vi "test_riccat_01i.vi"() -> (3 "All Tests Passed":bool)   [LabVIEW 2019]
uses:
  <vilib>/Analysis/Matrix/Datatypes/RealMatrix.ctl
  <vilib>/Rock Robotics/WPI/ThirdParty/JAS_Junk/TrajLib/Trajectory_Library.lvlib
  <vilib>/Analysis/Matrix/NI_Matrix.lvlib
panel:
  out "Eigenvalues":cdb[](array[numeric])
  out "error out":errorcluster
  out "Error":bool
  out "Iterations":i32
  out "Elapsed \nTime MS":dbl
  out "ZERO":T1
  out "X  Answer":T1
  in  "R":T1=[[0.25]]
  in  "Q":T1=[[1.0, 0.0, 0.0, 0.0], [0.0, 0.0, 0.0, 0.0], [0.0, 0.0, 0.0, 0.0], [0.0, 0.0, 0.0, 0.0]]
  in  "B":T1=[[0.0], [0.0], [0.0], [1.0]]
  in  "A":T1=[[0.5, 1.0, 0.0, 0.0], [0.0, 0.0, 1.0, 0.0], [0.0, 0.0, 0.0, 1.0], [0.0, 0.0, 0.0, 0.0]]
  # "Test 1: non-invertible A\n  // Example 2 of \"On the Numerical Solution of the Discrete-Time Algebraic\n  // Riccati Equation\""
  # "int n1 = 4, m1 = 1;"
  # "Example = F"
  # "MatrixXd A1(n1, n1), B1(n1, m1), Q1(n1, n1), R1(m1, m1);"
  # "A1 << 0.5, 1, 0, 0, \n          0, 0, 1, 0, \n          0, 0, 0, 1, \n          0, 0, 0, 0;"
  # "B1 << 0, \n        0, \n        0, \n        1;"
  # "Example G1"
  # "Example H"
  # "Solution weight ??"
  # "Q1 << 1, 0, 0, 0, \n        0, 0, 0, 0, \n        0, 0, 0, 0, \n        0, 0, 0, 0;"
  # "Example G2"
  # "Cost ??"
  # "R1 << 0.25;"
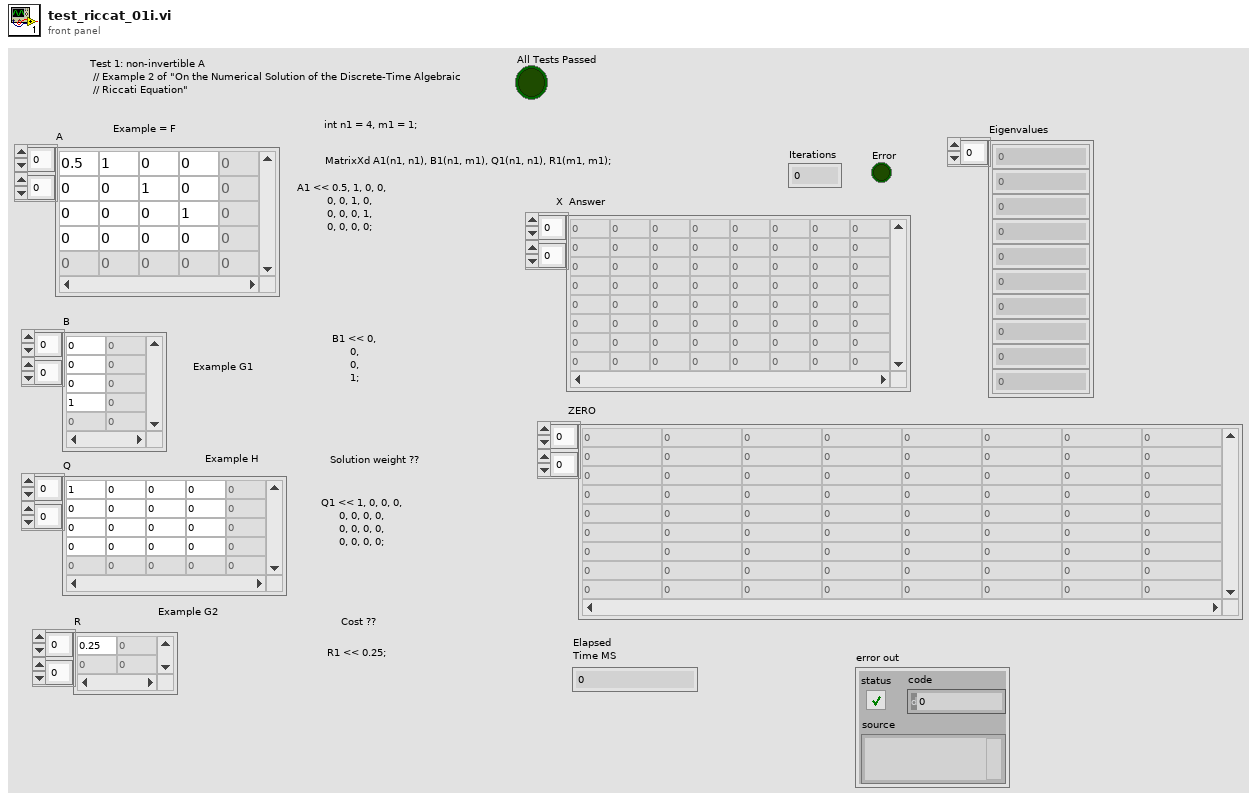
[diagram p1: front panel]
types:
  T1 = typedef "NI_Matrix.lvlib/RealMatrix.ctl" = dbl[][]
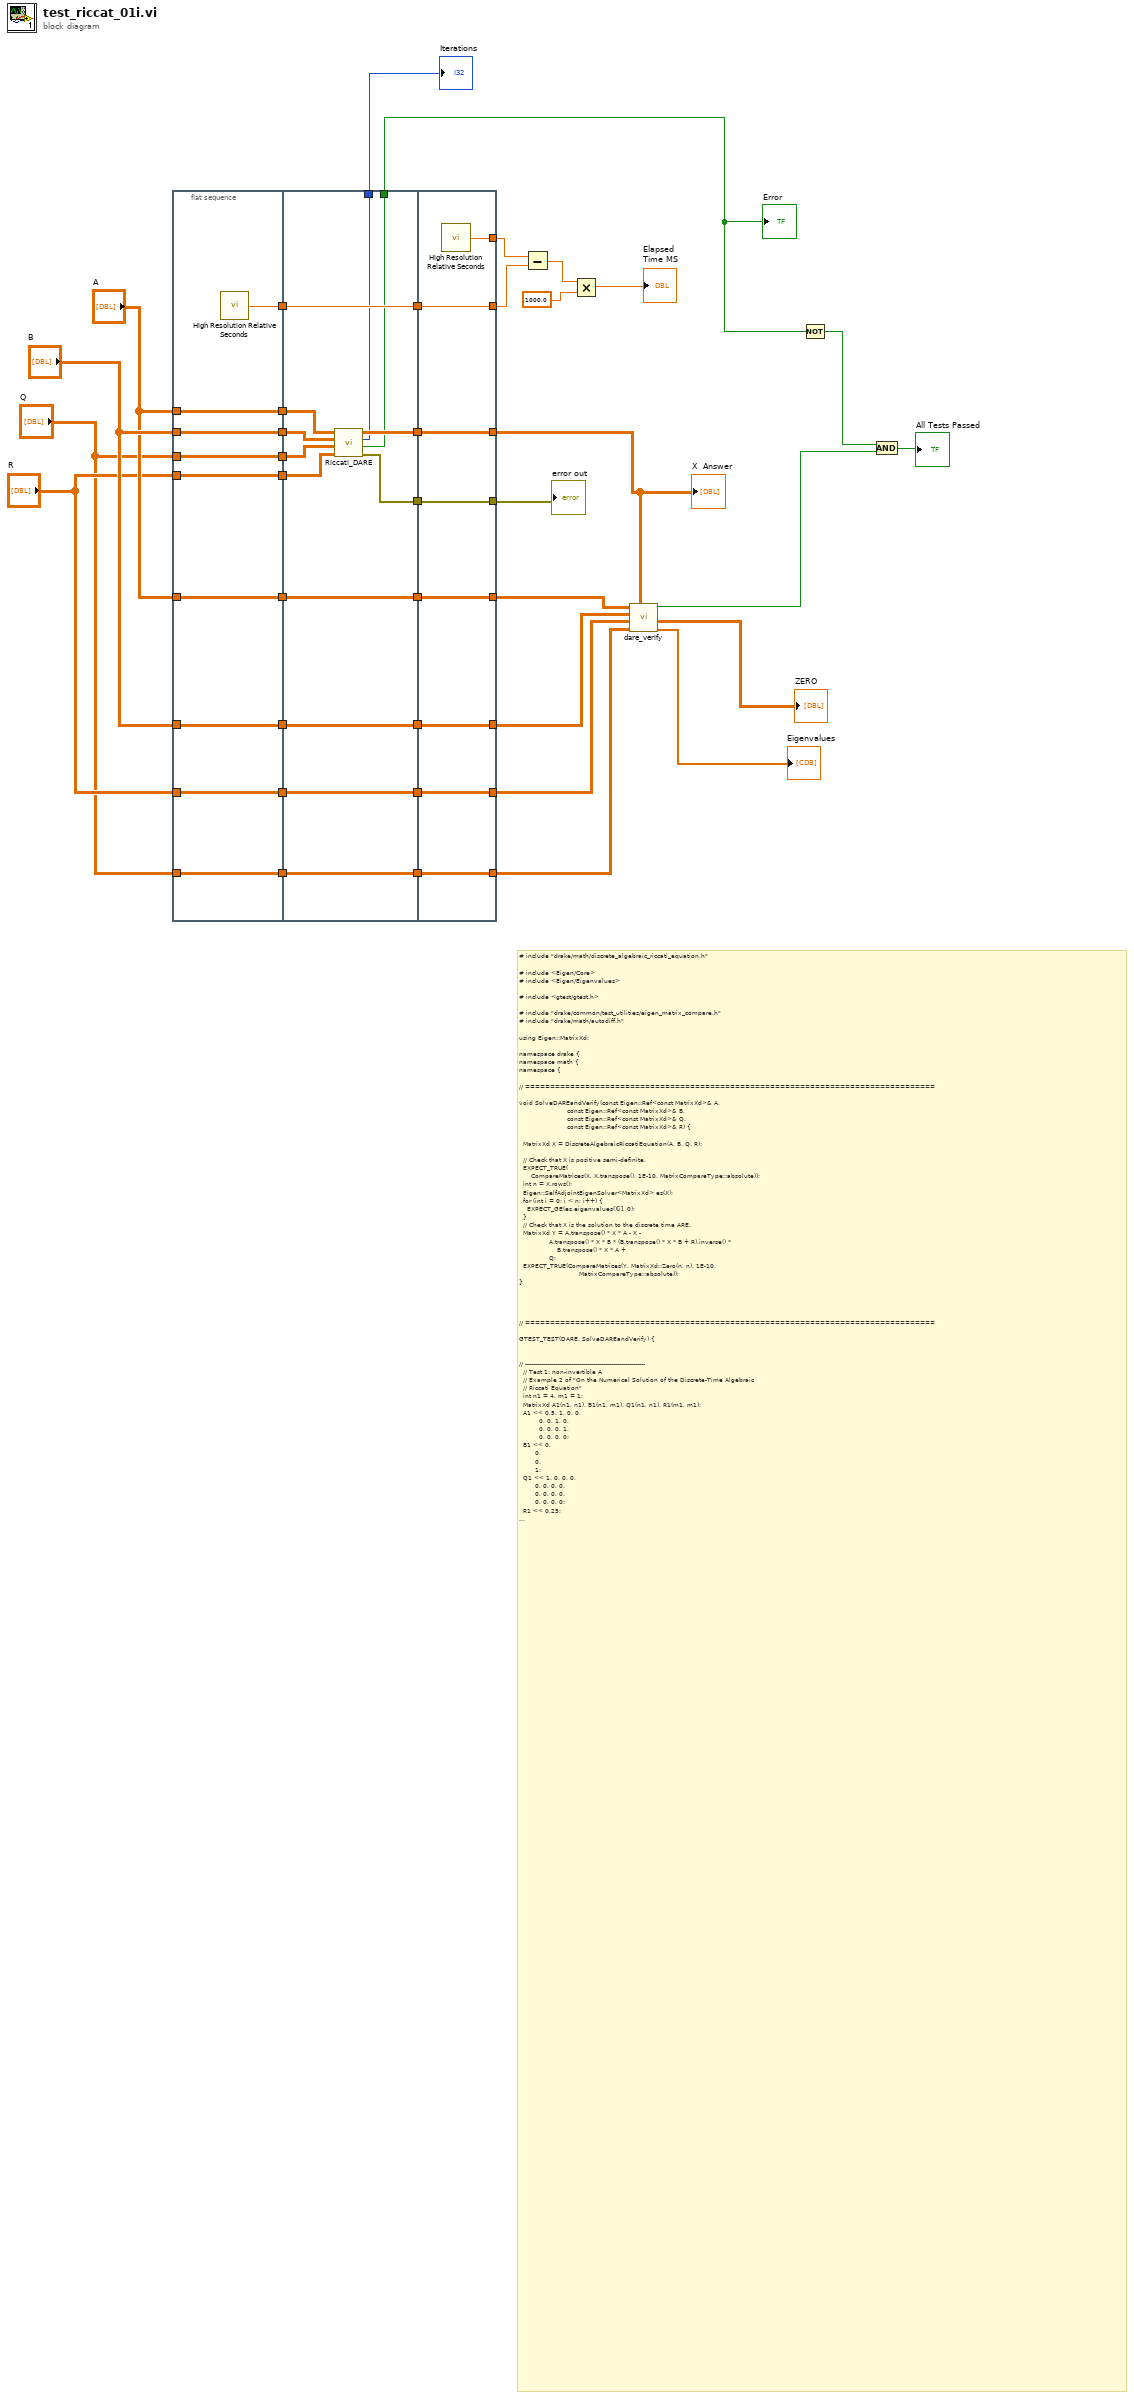
[diagram p0: block diagram]
diagram:
  # "# include \"drake/math/discrete_algebraic_riccati_equation.h\"\n\n# include <Eigen/Core>\n# include <Eigen/Eigenvalues>\n\n# include <gtest/gtest.h>\n\n# include \"drake/common/test_utilities/eigen_matrix_compare.h\"\n# include \"drake/math/autodiff.h\"\n\nusing Eigen::MatrixXd;\n\nnamespace drake {\nnamespace math {\nnamespace {\n\n// ==================================================================================\n\nvoid SolveDAREandVerify(const Eigen::Ref<const MatrixXd>& A,\n                        const Eigen::Ref<const MatrixXd>& B,\n                        const Eigen::Ref<const MatrixXd>& Q,\n                        const Eigen::Ref<const MatrixXd>& R) {\n\n  MatrixXd X = DiscreteAlgebraicRiccatiEquation(A, B, Q, R);\n\n  // Check that X is positive semi-definite.\n  EXPECT_TRUE(\n      CompareMatrices(X, X.transpose(), 1E-10, MatrixCompareType::absolute));\n  int n = X.rows();\n  Eigen::SelfAdjointEigenSolver<MatrixXd> es(X);\n  for (int i = 0; i < n; i++) {\n    EXPECT_GE(es.eigenvalues()[i], 0);\n  }\n  // Check that X is the solution to the discrete time ARE.\n  MatrixXd Y = A.transpose() * X * A - X -\n               A.transpose() * X * B * (B.transpose() * X * B + R).inverse() *\n                   B.transpose() * X * A +\n               Q;\n  EXPECT_TRUE(CompareMatrices(Y, MatrixXd::Zero(n, n), 1E-10,\n                              MatrixCompareType::absolute));\n}\n\n\n\n\n// ==================================================================================\n\nGTEST_TEST(DARE, SolveDAREandVerify) {\n\n\n// ------------------------------------------------------------\n  // Test 1: non-invertible A\n  // Example 2 of \"On the Numerical Solution of the Discrete-Time Algebraic\n  // Riccati Equation\"\n  int n1 = 4, m1 = 1;\n  MatrixXd A1(n1, n1), B1(n1, m1), Q1(n1, n1), R1(m1, m1);\n  A1 << 0.5, 1, 0, 0, \n          0, 0, 1, 0, \n          0, 0, 0, 1, \n          0, 0, 0, 0;\n  B1 << 0, \n        0, \n        0, \n        1;\n  Q1 << 1, 0, 0, 0, \n        0, 0, 0, 0, \n        0, 0, 0, 0, \n        0, 0, 0, 0;\n  R1 << 0.25;\n  SolveDAREandVerify(A1, B1, Q1, R1);\n// ------------------------------------------------------------\n  // Test 2: invertible A\n  int n2 = 2, m2 = 1;\n  MatrixXd A2(n2, n2), B2(n2, m2), Q2(n2, n2), R2(m2, m2);\n  A2 << 1, 1, 0, 1;\n  B2 << 0, 1;\n  Q2 << 1, 0, 0, 0;\n  R2 << 0.3;\n  SolveDAREandVerify(A2, B2, Q2, R2);\n\n// ------------------------------------------------------------\n  // Test 3: the first generalized eigenvalue of (S,T) is stable\n  int n3 = 2, m3 = 1;\n  MatrixXd A3(n3, n3), B3(n3, m3), Q3(n3, n3), R3(m3, m3);\n  A3 << 0, 1, 0, 0;\n  B3 << 0, 1;\n  Q3 << 1, 0, 0, 1;\n  R3 << 1;\n  SolveDAREandVerify(A3, B3, Q3, R3);\n\n// ------------------------------------------------------------\n  // Test 4: A = B = Q = R = I_2 (2-by-2 identity matrix)\n  int n4 = 2, m4 = 2;\n  MatrixXd A4(n4, n4), B4(n4, m4), Q4(n4, n4), R4(m4, m4);\n  A4 << 1, 0, 0, 1;\n  B4 << 1, 0, 0, 1;\n  Q4 << 1, 0, 0, 1;\n  R4 << 1, 0, 0, 1;\n  SolveDAREandVerify(A4, B4, Q4, R4);\n\n// ------------------------------------------------------------\n}\n}  // namespace\n}  // namespace math\n}  // namespace drake"
  n1 = flat-sequence {
    tunnel: "B" -> [w42]
    tunnel: "A" -> [w43]
    tunnel: "B" -> [w44]
    tunnel: "Q" -> [w45]
    tunnel: "A" -> [w46]
    tunnel: "R" -> [w47]
    tunnel: [w47] -> w38
    tunnel: [w46] -> w37
    tunnel: [w45] -> w36
    tunnel: [w44] -> w35
    tunnel: [w43] -> w34
    tunnel: [w42] -> w33
    tunnel: "R" -> [w41]
    tunnel: [w41] -> w26
    tunnel: "Q" -> [w40]
    tunnel: [w40] -> w24
    tunnel: [w39] -> w18
    tunnel: w38 -> [w60]
    tunnel: w37 -> [w58]
    tunnel: w36 -> [w57]
    tunnel: w35 -> [w56]
    tunnel: w34 -> [w55]
    tunnel: w33 -> [w54]
    tunnel: [w59] -> w32
    tunnel: [w55] -> w31
    tunnel: [w54] -> w30
    tunnel: [w53] -> w27
    tunnel: w26 -> [w53]
    tunnel: w24 -> [w52]
    tunnel: [w52] -> w23
    tunnel: [w51] -> w19
    tunnel: w18 -> [w51]
    tunnel: [w50] -> w14
    tunnel: [w49] -> w13
    tunnel: [w48] -> w12
    tunnel: [w66] -> w8
    tunnel: [w67] -> w9
    tunnel: [w68] -> w10
    tunnel: w32 -> [w68]
    tunnel: w31 -> [w67]
    tunnel: w30 -> [w66]
    tunnel: [w65] -> w7
    tunnel: w27 -> [w65]
    tunnel: [w64] -> w6
    tunnel: w23 -> [w64]
    tunnel: [w63] -> w21
    tunnel: [w62] -> w20
    tunnel: w19 -> [w62]
    tunnel: w12 -> [w61]
    tunnel: [w61] -> w11
    frame #0 {
      n2 = call <vilib>:"High Resolution Relative Seconds.vi"() -> ("relative seconds"=w39:dbl)
    }
    frame #1 {
      n3 = call <vilib>:"Riccati_DARE.vi"("R"=w60, "Q"=w57, "B"=w56, "A"=w58) -> ("error out"=w48:errorcluster, "Error"=w49:bool, "Iterations"=w50:i32, "Answer"=w59:T1)  [unwired: 4 in]
    }
    frame #2 {
      n4 = call <vilib>:"High Resolution Relative Seconds.vi"() -> ("relative seconds"=w63:dbl)
    }
  }
  n5 = Subtract(x=w21, y=w20) -> (x-y=w17:dbl)
  n6 = Multiply(x=w17, y=1000.0) -> (x*y=→"Elapsed \nTime MS":dbl)
  n7 = call "dare_verify.vi"("Answer"=w10, "Q"=w6, "R"=w7, "B"=w8, "A"=w9) -> ("Eigenvalues"=→"Eigenvalues":cdb[], "ZERO"=→"ZERO":T1, "Passed"=w2:bool)  [unwired: 4 in]
  n8 = Not(x=w13) -> (.not. x?=w3:bool)
  n9 = And(x=w3, y=w2) -> (x .and. y?=→"All Tests Passed":bool)
  "X  Answer" <- w10
  "Iterations" <- w14
  "Error" <- w13
  "error out" <- w11
